vi "Windshield Wipers.vi"() -> ()   [LabVIEW 2013]
panel:
  out "Elapsed Time Text":string
  out "Time has Elapsed":bool
  in  "Automatic Timer Control\n(seconds)":dbl
  out "End Position":bool
  in  "Current State":enum16{"Stop", "Automatic", "Manual"}(ring)
  in  "Stop Button":bool
  out "Start Position":bool
  out "Manual":bool
  out "Automatic":bool
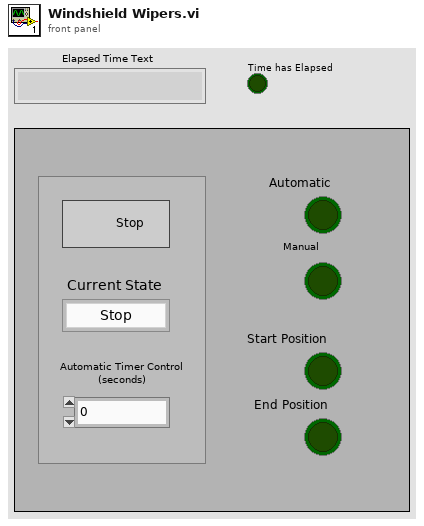
[diagram p1: front panel]
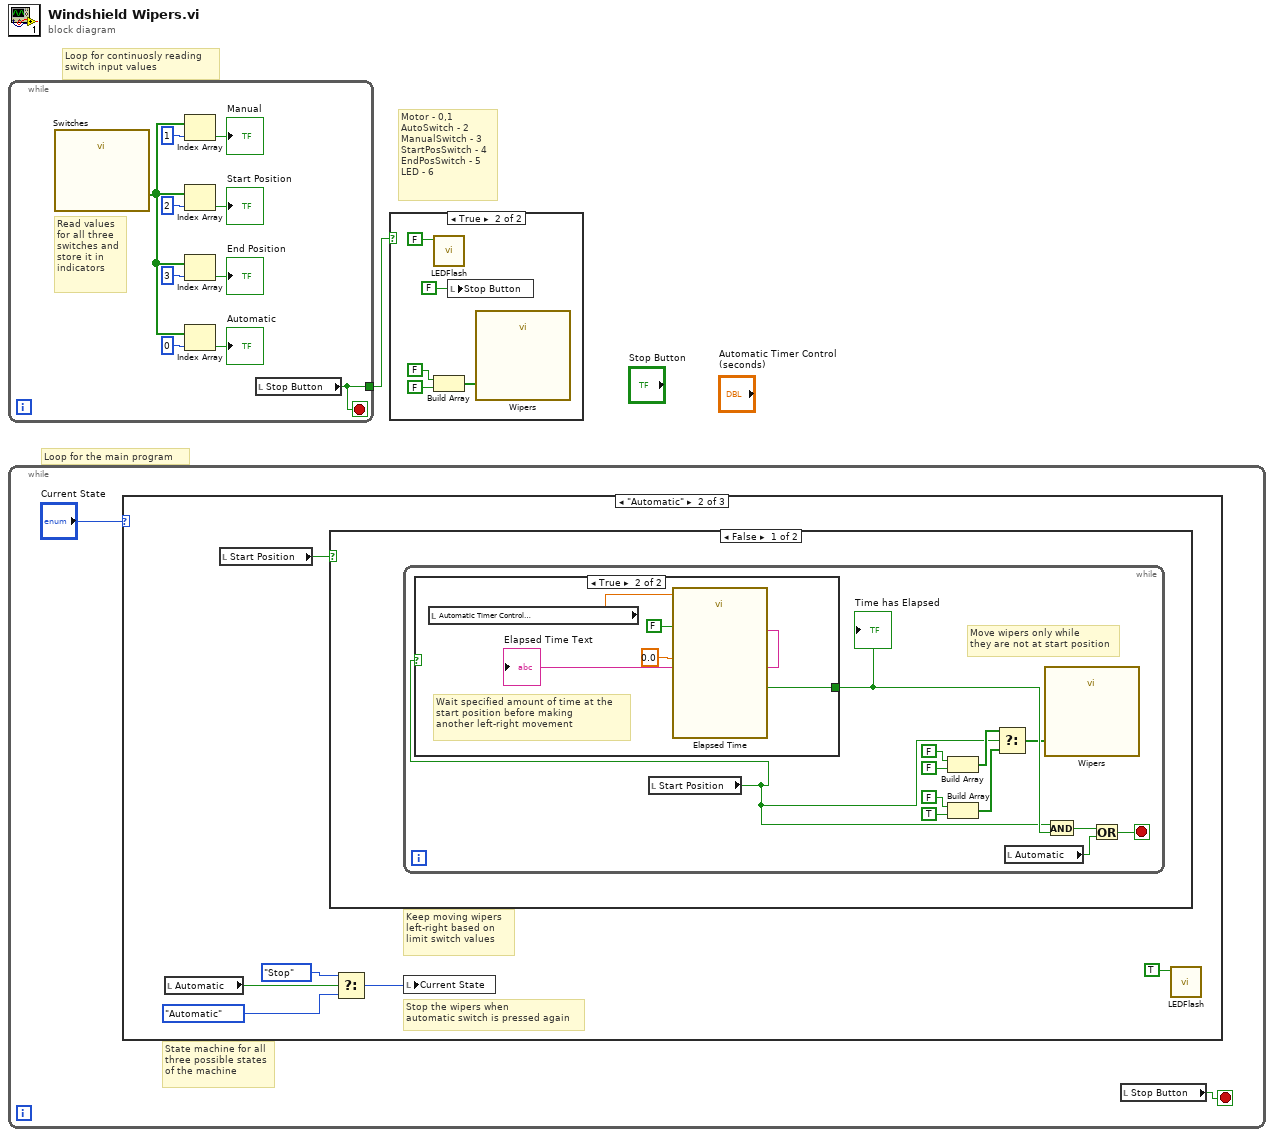
[diagram p0: block diagram]
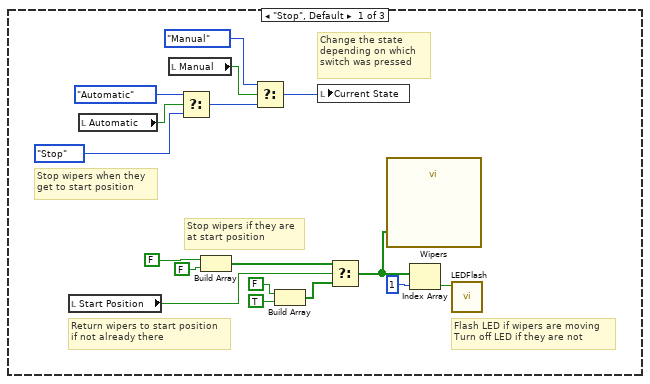
[diagram p3: hidden frame]
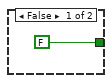
[diagram p4: hidden frame]
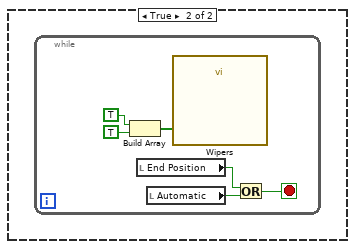
[diagram p5: hidden frame]
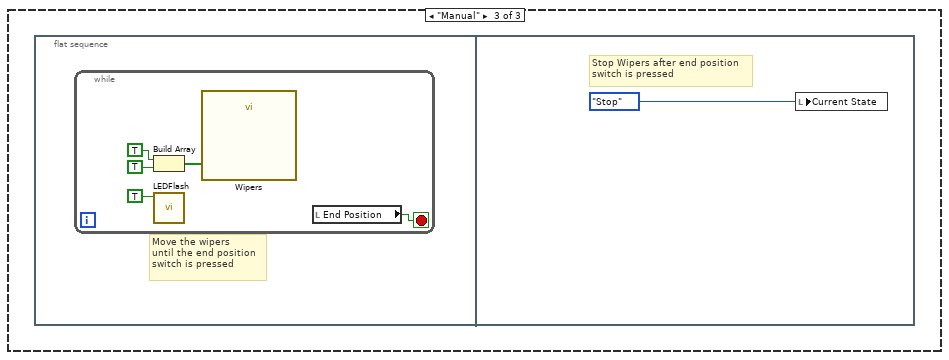
[diagram p6: hidden frame]
diagram:
  # "Loop for the main program"
  # "Loop for continuosly reading\nswitch input values"
  # "Motor - 0,1\nAutoSwitch - 2\nManualSwitch - 3\nStartPosSwitch - 4\nEndPosSwitch - 5\nLED - 6"
  n1 = while {
    tunnel: [w2] -> w1
    stop <- w2 stop-if-true
    # "Read values\nfor all three\nswitches and\nstore it in \nindicators"
    n2 = call "Switches"() -> ("data"=w4:bool[])  [unwired: 17 in, 2 out]
    n3 = Index Array(array=w4, index=1) -> (element=→"Manual":bool)
    n4 = Index Array(array=w4, index=2) -> (element=→"Start Position":bool)
    n5 = Index Array(array=w4, index=3) -> (element=→"End Position":bool)
    n6 = Index Array(array=w4, index=0) -> (element=→"Automatic":bool)
    n7 = local read "Stop Button"() -> (w2:bool)
  }
  n8 = while {
    stop <- w13 stop-if-true
    # "State machine for all\nthree possible states\nof the machine"
    n9 = case shown="\"Automatic\"" "Current State" {
      frame "Stop", Default {
        # "Stop wipers if they are\nat start position"
        # "Flash LED if wipers are moving\nTurn off LED if they are not"
        # "Stop wipers when they\nget to start position"
        # "Return wipers to start position\nif not already there"
        # "Change the state\ndepending on which\nswitch was pressed"
        n10 = local read "Start Position"() -> (w21:bool)
        n11 = local read "Automatic"() -> (w27:bool)
        n12 = local read "Manual"() -> (w28:bool)
        n13 = Select(t=enum16{"Stop", "Automatic", "Manual"}."Automatic" ("Current State"), s=w27, f=enum16{"Stop", "Automatic", "Manual"}."Stop" ("Current State")) -> (s? t:f=w22:enum16{"Stop", "Automatic", "Manual"})
        n14 = Build Array(FALSE, FALSE) -> (w20:bool[])
        n15 = Select(t=enum16{"Stop", "Automatic", "Manual"}."Manual" ("Current State"), s=w28, f=w22) -> (s? t:f=w25:enum16{"Stop", "Automatic", "Manual"})
        n16 = Build Array(FALSE, TRUE) -> (w17:bool[])
        n17 = local write "Current State"(w25) -> ()
        n18 = Select(t=w20, s=w21, f=w17) -> (s? t:f=w16:bool[])
        n19 = call "Wipers"("data"=w16) -> ()  [unwired: 17 in, 2 out]
        n20 = Index Array(array=w16, index=1) -> (element=w14:bool)
        n21 = call "LEDFlash.vi"("Boolean"=w14) -> ()  [unwired: 11 in]
      }
      frame "Automatic" {
        # "Keep moving wipers\nleft-right based on\nlimit switch values"
        # "Stop the wipers when\nautomatic switch is pressed again"
        n22 = local read "Automatic"() -> (w35:bool)
        n23 = local read "Start Position"() -> (w36:bool)
        n24 = case shown="False" w36 {
          frame False {
            n25 = while {
              stop <- w45 stop-if-true
              # "Move wipers only while\nthey are not at start position"
              n26 = local read "Start Position"() -> (w37:bool)
              n27 = case shown="True" w37 {
                tunnel: [FALSE ("Time has Elapsed") w54] -> w44
                frame False {
                }
                frame True {
                  # "Wait specified amount of time at the\nstart position before making\nanother left-right movement"
                  n28 = local read "Automatic Timer Control\n(seconds)"() -> (w53:dbl)
                  n29 = call "Elapsed Time"("Time Target (s)"=w53, "Auto Reset"=FALSE, "Set Start Time (s)"=0.0) -> ("Time has Elapsed"=w54:bool, "Elapsed Time Text"=→"Elapsed Time Text":string)  [unwired: 9 in, 6 out]
                }
              }
              "Time has Elapsed" <- w44
              n30 = Build Array(FALSE, FALSE) -> (w39:bool[])
              n31 = Build Array(FALSE, TRUE) -> (w42:bool[])
              n32 = Select(t=w39, s=w37, f=w42) -> (s? t:f=w38:bool[])
              n33 = local read "Automatic"() -> (w46:bool)
              n34 = call "Wipers"("data"=w38) -> ()  [unwired: 17 in, 2 out]
              n35 = And(x=w37, y=w44) -> (x .and. y?=w43:bool)
              n36 = Or(x=w43, y=w46) -> (x .or. y?=w45:bool)
            }
          }
          frame True {
            n37 = while {
              stop <- w55 stop-if-true
              n38 = Build Array(TRUE, TRUE) -> (w58:bool[])
              n39 = local read "End Position"() -> (w57:bool)
              n40 = local read "Automatic"() -> (w56:bool)
              n41 = call "Wipers"("data"=w58) -> ()  [unwired: 17 in, 2 out]
              n42 = Or(x=w57, y=w56) -> (x .or. y?=w55:bool)
            }
          }
        }
        n43 = Select(t=enum16{"Stop", "Automatic", "Manual"}."Stop" ("Current State"), s=w35, f=enum16{"Stop", "Automatic", "Manual"}."Automatic" ("Current State")) -> (s? t:f=w33:enum16{"Stop", "Automatic", "Manual"})
        n44 = local write "Current State"(w33) -> ()
        n45 = call "LEDFlash.vi"("Boolean"=TRUE) -> ()  [unwired: 11 in]
      }
      frame "Manual" {
        n46 = flat-sequence {
          frame #0 {
            # "Move the wipers\nuntil the end position\nswitch is pressed"
            n47 = while {
              stop <- w62 stop-if-true
              n48 = Build Array(TRUE, TRUE) -> (w63:bool[])
              n49 = call "LEDFlash.vi"("Boolean"=TRUE) -> ()  [unwired: 11 in]
              n50 = call "Wipers"("data"=w63) -> ()  [unwired: 17 in, 2 out]
              n51 = local read "End Position"() -> (w62:bool)
            }
          }
          frame #1 {
            # "Stop Wipers after end position\nswitch is pressed"
            n52 = local write "Current State"(enum16{"Stop", "Automatic", "Manual"}."Stop" ("Current State")) -> ()
          }
        }
      }
    }
    n53 = local read "Stop Button"() -> (w13:bool)
  }
  n54 = case shown="True" w1 {
    frame False {
    }
    frame True {
      n55 = call "LEDFlash.vi"("Boolean"=FALSE) -> ()  [unwired: 11 in]
      n56 = Build Array(FALSE, FALSE) -> (w68:bool[])
      n57 = local write "Stop Button"(FALSE ("Stop Button")) -> ()
      n58 = call "Wipers"("data"=w68) -> ()  [unwired: 17 in, 2 out]
    }
  }
